vi "asset.create.vi"(8 "error in":errorcluster, 9 "Description":string, 10 "Title":string, 11 "Nominal Client in":refnum<class "Nominal Client.lvclass">) -> (0 "error out":errorcluster, 2 "asset":refnum<class "asset.lvclass">, 3 "Nominal Client out":refnum<class "Nominal Client.lvclass">)   [LabVIEW 2020, in "Nominal Client.lvclass"]
doc: "Triggers an ingest job, allowing either creating a new dataset or uploading to an existing one. This endpoint is meant to supersede all other ingestion endpoints as their functionality gets migrated to this one."
uses:
  Nominal Client.lvclass
  asset/asset.lvclass
  Nominal Client.lvclass/Nominal Client.ctl
  nominal types/workspace/workspace.lvclass/workspace.ctl
  ece5603b-f0cd-498c-a843-52d0aa39fd1b.vi
  828a30e2-c590-4274-9f47-5329aaebfb4a.vi
  workspace.get.vi
  <vilib>/JDP Science/JSONtext/Merge into Object.vi
  workspace.add_to_payload.vi/88650e10-de3e-481c-85db-71cb0fdf4485.vi
  nominal types/workspace/rid.get.vi
  <vilib>/JDP Science/JSONtext/Variant to JSON Text.vi
  <vilib>/JDP Science/JSONtext/Get all Object Items.vi
  <vilib>/JDP Science/JSONtext/Set Multiple Object Items.vi
  <vilib>/JDP Science/JSONtext/LVClass Serializer/JSONtext LVClass Serializer.lvclass
  <vilib>/JDP Science/JSONtext/JSONtext.lvlib
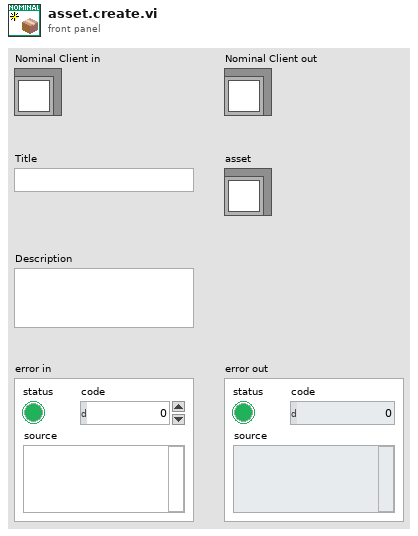
[diagram p1: front panel]
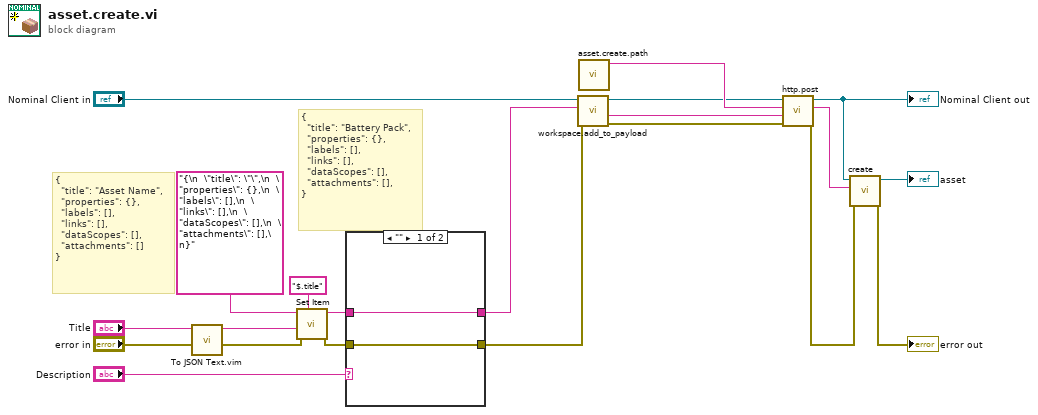
[diagram p0: block diagram]
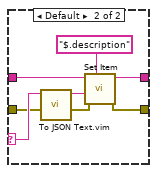
[diagram p2: hidden frame]
diagram:
  # "{\n  \"title\": \"Battery Pack\",\n  \"properties\": {},\n  \"labels\": [],\n  \"links\": [],\n  \"dataScopes\": [],\n  \"attachments\": [],\n}"
  # "{\n  \"title\": \"Asset Name\",\n  \"properties\": {},\n  \"labels\": [],\n  \"links\": [],\n  \"dataScopes\": [],\n  \"attachments\": []\n}"
  n1 = call "To JSON Text.vim"("error in (no error)"="error in", "Anything"="Title") -> ("error out"=w17:errorcluster, "<JSON>"=w19:string)  [unwired: 8 in]
  n2 = call <vilib>:"Set Item.vi"("$Path or Item Name"="$.title", "error in (no error)"=w17, "JSON to Insert"=w19, "JSON"="{\n  \"title\": \"\",\n  \"properties\": {},\n  \"labels\": [],\n  \"links\": [],\n  \"dataScopes\": [],\n  \"attachments\": [],\n}") -> ("error out"=w16:errorcluster, "<JSON>"=w18:string)  [unwired: 4 in, 1 out]
  n3 = case shown="\"\"" "Description" {
    selector: "Description" -> [_ w29]
    tunnel: w18 -> [w23 w30]
    tunnel: [w23 w27] -> w6
    tunnel: w16 -> [w22 w26]
    tunnel: [w22 w24] -> w1
    frame "" {
    }
    frame Default {
      n4 = call "To JSON Text.vim"("error in (no error)"=w26, "Anything"=w29) -> ("error out"=w25:errorcluster, "<JSON>"=w28:string)  [unwired: 8 in]
      n5 = call <vilib>:"Set Item.vi"("$Path or Item Name"="$.description", "error in (no error)"=w25, "JSON to Insert"=w28, "JSON"=w30) -> ("error out"=w24:errorcluster, "<JSON>"=w27:string)  [unwired: 4 in, 1 out]
    }
  }
  n6 = call "workspace.add_to_payload.vi"("error in"=w1, "JSON payload in"=w6, "Nominal Client in"="Nominal Client in") -> ("error out"=w4:errorcluster, "JSON payload out"=w5:string, "Nominal Client out"=w3:refnum<class "Nominal Client.lvclass">)  [unwired: 6 in]
  n7 = call "asset.create.path.vi"() -> ("path"=w7:string)  [unwired: 10 in, 1 out]
  n8 = call "http.post.vi"("error in"=w4, "Request body"=w5, "Path"=w7, "Nominal Client in"=w3) -> ("error out"=w11:errorcluster, "Response"=w12:string, "Nominal Client out"=w8:refnum<class "Nominal Client.lvclass">)  [unwired: 4 in, 1 out]
  "Nominal Client out" <- w8
  n9 = call "create.vi"("error in"=w11, "asset"=w12, "Nominal Client"=w8) -> ("error out"=→"error out":errorcluster, "asset"=→"asset":refnum<class "asset.lvclass">)  [unwired: 7 in]
